vi "Read Dashboard Variables.vi"() -> ()   [LabVIEW 2019]
uses:
  <vilib>/Rock Robotics/Network Tables/NT Read Number.vi
  Framework/Robot Global Data.vi
  <vilib>/Rock Robotics/Network Tables/NT Read String.vi
panel:
  out "Limelight search speed":dbl=0.3 min=0.0 max=1.0 step=0.1
  out "Pivot Increase":dbl min=0.0 max=0.5 step=0.1
  out "MaxSpeedSlow Bumps":dbl=0.6
  out "Shooter Set Point Low Target":dbl=1.0
  out "Path":string
  out "MaxSpeedSlow":dbl=0.6
  out "Pivot Left":dbl=0.3
  out "Pivot right":dbl=0.4
  out "Intake Set Point":dbl=1.0
  out "Intake Duration":dbl=0.5
  out "Shooter Set Point":dbl=1.0
  out "Shooter Duration":dbl=0.5
  out "Transfer Set Point":dbl=0.6
  out "Transfer Duration":dbl=0.5
  out "Control Panel Set Point":dbl=0.6
  out "Control Panel Duration":dbl=5.5
  out "Control Panel Color Set Point":dbl=0.3
  out "Control Panel Color Duration":dbl=4.0
  out "MaxDrive":dbl(slide)=1.0 min=0.0 max=1.0 step=0.01 scale=0.0..1.0
  out "DriveK":dbl(slide)=0.5 min=0.0 max=1.0 step=0.05 scale=0.0..1.0
  out "Limelight Goal Area":dbl(slide)=1.91 min=0.1 max=2.5 step=0.25 scale=0.0..2.5
  out "MinSteerCommand":dbl(slide)=0.2717391304347826 min=0.0 max=0.5 step=0.05 scale=0.0..0.5
  out "SteeringK":dbl(slide)=0.025362318840579712 min=0.0 max=0.25 step=0.01 scale=0.0..0.25
  out "AimDeadband":dbl=0.1 min=0.0 max=10.0 step=0.25
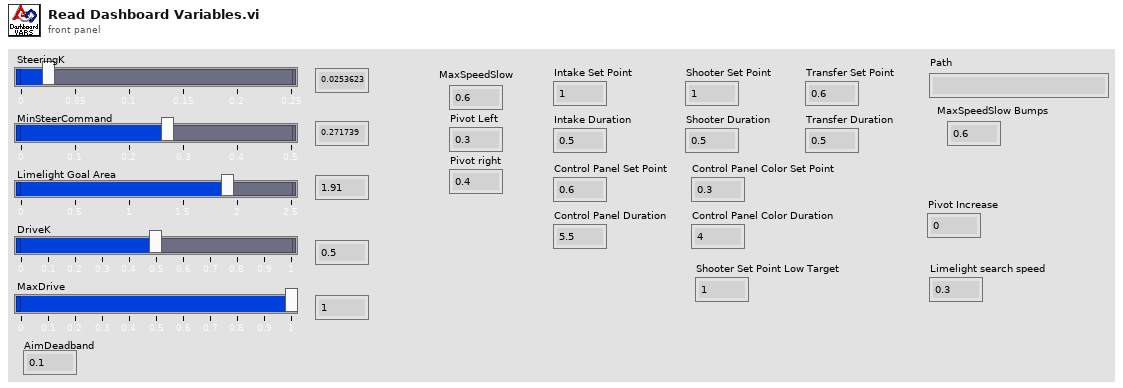
[diagram p1: front panel]
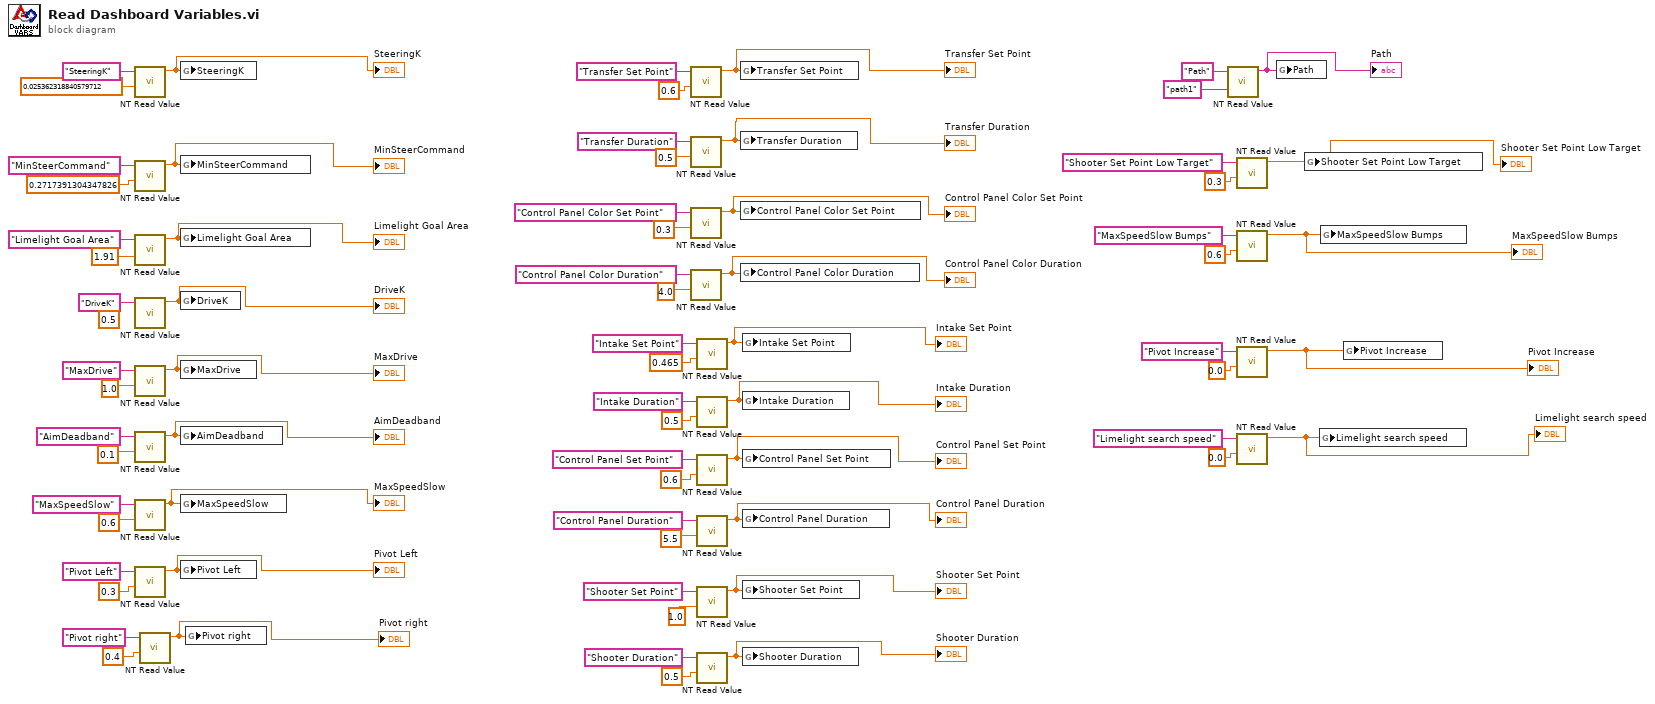
[diagram p0: block diagram]
diagram:
  (unwired) 0.5 ("DriveK")
  n1 = call-poly <vilib>:"NT Read Value.vi"("Default Value"=0.025362318840579712 ("SteeringK"), "Name"="SteeringK") -> ("Numeric"=w34:dbl)  [unwired: 8 in, 1 out]
  "SteeringK" <- w34
  n2 = call-poly <vilib>:"NT Read Value.vi"("Default Value"=0.2717391304347826 ("MinSteerCommand"), "Name"="MinSteerCommand") -> ("Numeric"=w17:dbl)  [unwired: 8 in, 1 out]
  "MinSteerCommand" <- w17
  n3 = call-poly <vilib>:"NT Read Value.vi"("Default Value"=1.91 ("Limelight Goal Area"), "Name"="Limelight Goal Area") -> ("Numeric"=w33:dbl)  [unwired: 8 in, 1 out]
  "Limelight Goal Area" <- w33
  n4 = call-poly <vilib>:"NT Read Value.vi"("Name"="DriveK") -> ("Numeric"=w32:dbl)  [unwired: 9 in, 1 out]
  "DriveK" <- w32
  n5 = call-poly <vilib>:"NT Read Value.vi"("Default Value"=1.0 ("MaxDrive"), "Name"="MaxDrive") -> ("Numeric"=w31:dbl)  [unwired: 8 in, 1 out]
  "MaxDrive" <- w31
  n6 = call-poly <vilib>:"NT Read Value.vi"("Default Value"=0.1 ("AimDeadband"), "Name"="AimDeadband") -> ("Numeric"=w30:dbl)  [unwired: 8 in, 1 out]
  "AimDeadband" <- w30
  n7 = call-poly <vilib>:"NT Read Value.vi"("Default Value"=0.6 ("MaxSpeedSlow"), "Name"="MaxSpeedSlow") -> ("Numeric"=w29:dbl)  [unwired: 8 in, 1 out]
  "MaxSpeedSlow" <- w29
  n8 = call-poly <vilib>:"NT Read Value.vi"("Default Value"=0.3 ("Pivot Left"), "Name"="Pivot Left") -> ("Numeric"=w28:dbl)  [unwired: 8 in, 1 out]
  "Pivot Left" <- w28
  n9 = call-poly <vilib>:"NT Read Value.vi"("Default Value"=0.4 ("Pivot right"), "Name"="Pivot right") -> ("Numeric"=w27:dbl)  [unwired: 8 in, 1 out]
  "Pivot right" <- w27
  n10 = global write "Robot Global Data.vi" "SteeringK"(w34) -> ()
  n11 = global write "Robot Global Data.vi" "MinSteerCommand"(w17) -> ()
  n12 = global write "Robot Global Data.vi" "Limelight Goal Area"(w33) -> ()
  n13 = global write "Robot Global Data.vi" "DriveK"(w32) -> ()
  n14 = global write "Robot Global Data.vi" "MaxDrive"(w31) -> ()
  n15 = global write "Robot Global Data.vi" "AimDeadband"(w30) -> ()
  n16 = global write "Robot Global Data.vi" "MaxSpeedSlow"(w29) -> ()
  n17 = global write "Robot Global Data.vi" "Pivot Left"(w28) -> ()
  n18 = global write "Robot Global Data.vi" "Pivot right"(w27) -> ()
  n19 = call-poly <vilib>:"NT Read Value.vi"("Default Value"=0.6 ("Transfer Set Point"), "Name"="Transfer Set Point") -> ("Numeric"=w21:dbl)  [unwired: 8 in, 1 out]
  "Transfer Set Point" <- w21
  n20 = call-poly <vilib>:"NT Read Value.vi"("Default Value"=0.5 ("Transfer Duration"), "Name"="Transfer Duration") -> ("Numeric"=w20:dbl)  [unwired: 8 in, 1 out]
  "Transfer Duration" <- w20
  n21 = call-poly <vilib>:"NT Read Value.vi"("Default Value"=0.3 ("Control Panel Color Set Point"), "Name"="Control Panel Color Set Point") -> ("Numeric"=w19:dbl)  [unwired: 8 in, 1 out]
  "Control Panel Color Set Point" <- w19
  n22 = call-poly <vilib>:"NT Read Value.vi"("Default Value"=4.0 ("Control Panel Color Duration"), "Name"="Control Panel Color Duration") -> ("Numeric"=w18:dbl)  [unwired: 8 in, 1 out]
  "Control Panel Color Duration" <- w18
  n23 = call-poly <vilib>:"NT Read Value.vi"("Default Value"=0.465 ("Intake Set Point"), "Name"="Intake Set Point") -> ("Numeric"=w16:dbl)  [unwired: 8 in, 1 out]
  "Intake Set Point" <- w16
  n24 = call-poly <vilib>:"NT Read Value.vi"("Default Value"=0.5 ("Intake Duration"), "Name"="Intake Duration") -> ("Numeric"=w26:dbl)  [unwired: 8 in, 1 out]
  "Intake Duration" <- w26
  n25 = call-poly <vilib>:"NT Read Value.vi"("Default Value"=0.6 ("Control Panel Set Point"), "Name"="Control Panel Set Point") -> ("Numeric"=w25:dbl)  [unwired: 8 in, 1 out]
  "Control Panel Set Point" <- w25
  n26 = call-poly <vilib>:"NT Read Value.vi"("Default Value"=5.5 ("Control Panel Duration"), "Name"="Control Panel Duration") -> ("Numeric"=w24:dbl)  [unwired: 8 in, 1 out]
  "Control Panel Duration" <- w24
  n27 = call-poly <vilib>:"NT Read Value.vi"("Default Value"=1.0 ("Shooter Set Point"), "Name"="Shooter Set Point") -> ("Numeric"=w23:dbl)  [unwired: 8 in, 1 out]
  "Shooter Set Point" <- w23
  n28 = call-poly <vilib>:"NT Read Value.vi"("Default Value"=0.5 ("Shooter Duration"), "Name"="Shooter Duration") -> ("Numeric"=w22:dbl)  [unwired: 8 in, 1 out]
  "Shooter Duration" <- w22
  n29 = global write "Robot Global Data.vi" "Transfer Set Point"(w21) -> ()
  n30 = global write "Robot Global Data.vi" "Transfer Duration"(w20) -> ()
  n31 = global write "Robot Global Data.vi" "Control Panel Color Set Point"(w19) -> ()
  n32 = global write "Robot Global Data.vi" "Control Panel Color Duration"(w18) -> ()
  n33 = global write "Robot Global Data.vi" "Intake Set Point"(w16) -> ()
  n34 = global write "Robot Global Data.vi" "Intake Duration"(w26) -> ()
  n35 = global write "Robot Global Data.vi" "Control Panel Set Point"(w25) -> ()
  n36 = global write "Robot Global Data.vi" "Control Panel Duration"(w24) -> ()
  n37 = global write "Robot Global Data.vi" "Shooter Set Point"(w23) -> ()
  n38 = global write "Robot Global Data.vi" "Shooter Duration"(w22) -> ()
  n39 = call-poly <vilib>:"NT Read Value.vi"("Default Value"="path1", "Name"="Path") -> ("String"=w13:string)  [unwired: 8 in, 1 out]
  "Path" <- w13
  n40 = call-poly <vilib>:"NT Read Value.vi"("Default Value"=0.3 ("Transfer Set Point"), "Name"="Shooter Set Point Low Target") -> ("Numeric"=w10:dbl)  [unwired: 8 in, 1 out]
  "Shooter Set Point Low Target" <- w10
  n41 = call-poly <vilib>:"NT Read Value.vi"("Default Value"=0.6 ("Transfer Set Point"), "Name"="MaxSpeedSlow Bumps") -> ("Numeric"=w7:dbl)  [unwired: 8 in, 1 out]
  "MaxSpeedSlow Bumps" <- w7
  n42 = call-poly <vilib>:"NT Read Value.vi"("Default Value"=0.0 ("Transfer Set Point"), "Name"="Pivot Increase") -> ("Numeric"=w4:dbl)  [unwired: 8 in, 1 out]
  "Pivot Increase" <- w4
  n43 = call-poly <vilib>:"NT Read Value.vi"("Default Value"=0.0 ("Transfer Set Point"), "Name"="Limelight search speed") -> ("Numeric"=w1:dbl)  [unwired: 8 in, 1 out]
  "Limelight search speed" <- w1
  n44 = global write "Robot Global Data.vi" "Path"(w13) -> ()
  n45 = global write "Robot Global Data.vi" "Shooter Set Point Low Target"(w10) -> ()
  n46 = global write "Robot Global Data.vi" "Limelight search speed"(w1) -> ()
  n47 = global write "Robot Global Data.vi" "MaxSpeedSlow Bumps"(w7) -> ()
  n48 = global write "Robot Global Data.vi" "Pivot Increase"(w4) -> ()
